vi "Get Graph Data.vi"(0 "refresh time (ms)":i32, 1 "reading.var 1::1":dbl caption="Regen pulse energy" min=-100000.0 max=100000.0, 2 "Number of hours in buffer":dbl=96.0, 3 "MeanCounts::2":dbl caption="LM_Mirrorcam MeanCounts" min=0.0 max=999999999.0, 4 "MeanCounts::3":dbl caption="LM_Focuscam MeanCounts" min=0.0 max=999999999.0, 5 "MeanCounts::4":dbl caption="TS-253a_in MeanCounts" min=0.0 max=999999999.0, 6 "Data ip":T1) -> (14 "Data op":T1, 15 "Current array size":i32)   [LabVIEW 2013]
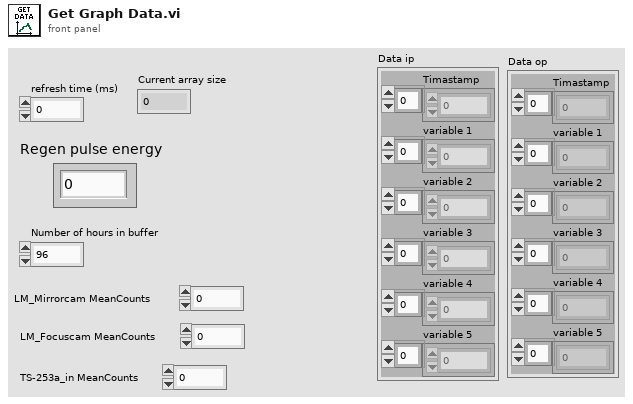
[diagram p1: front panel]
types:
  T1 = cluster{"Timastamp":dbl[], "variable 1":dbl[], "variable 2":dbl[], "variable 3":dbl[], "variable 4":dbl[], "variable 5":dbl[]}
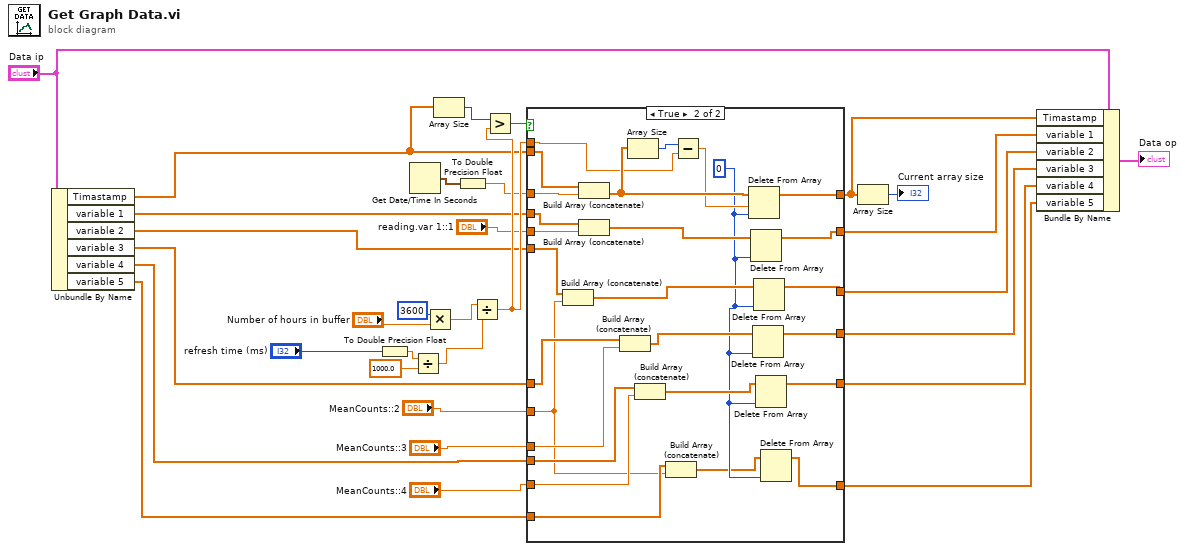
[diagram p0: block diagram]
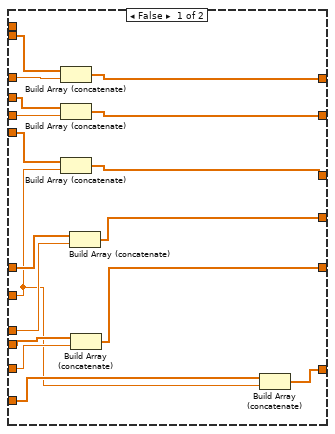
[diagram p2: hidden frame]
diagram:
  n1 = Unbundle By Name("Data ip") -> ("Timastamp"=w14:dbl[], "variable 1"=w13:dbl[], "variable 2"=w12:dbl[], "variable 3"=w11:dbl[], "variable 4"=w10:dbl[], "variable 5"=w9:dbl[])
  n2 = To Double Precision Float(number="refresh time (ms)") -> (double precision float=w22:dbl)
  n3 = Get Date/Time In Seconds() -> (seconds since 1Jan1904=w16:timestamp)
  n4 = Divide(x=w22, y=1000.0) -> (x/y=w26:dbl)
  n5 = Multiply(x=3600, y="Number of hours in buffer") -> (x*y=w25:dbl)
  n6 = Array Size(array=w14) -> (size(s)=w15:i32)
  n7 = To Double Precision Float(number=w16) -> (double precision float=w18:dbl)
  n8 = Divide(x=w25, y=w26) -> (x/y=w28:dbl)
  n9 = Greater?(x=w15, y=w28) -> (0:w17:bool)
  n10 = case shown="True" w17 {
    tunnel: w18 -> [w48 w75]
    tunnel: "reading.var 1::1" -> [w45 w74]
    tunnel: [w47 w70] -> w7
    tunnel: [w46 w69] -> w6
    tunnel: w14 -> [w44 w73]
    tunnel: w13 -> [w43 w72]
    tunnel: w28 -> [_ w66]
    tunnel: "MeanCounts::2" -> [w32 w49]
    tunnel: w12 -> [w42 w63]
    tunnel: [w41 w62] -> w5
    tunnel: "MeanCounts::3" -> [w38 w59]
    tunnel: "MeanCounts::4" -> [w34 w58]
    tunnel: [w40 w57] -> w4
    tunnel: [w39 w56] -> w3
    tunnel: w10 -> [w37 w55]
    tunnel: w11 -> [w36 w54]
    tunnel: w9 -> [w35 w50]
    tunnel: [w33 w52] -> w2
    frame False {
      n11 = Build Array (concatenate)(w44, w48) -> (w47:dbl[])
      n12 = Build Array (concatenate)(w43, w45) -> (w46:dbl[])
      n13 = Build Array (concatenate)(w42, w32) -> (w41:dbl[])
      n14 = Build Array (concatenate)(w36, w38) -> (w40:dbl[])
      n15 = Build Array (concatenate)(w37, w34) -> (w39:dbl[])
      n16 = Build Array (concatenate)(w35, w32) -> (w33:dbl[])
    }
    frame True {
      w53 = 0
      n17 = Build Array (concatenate)(w63, w49) -> (w64:dbl[])
      n18 = Build Array (concatenate)(w73, w75) -> (w68:dbl[])
      n19 = Build Array (concatenate)(w72, w74) -> (w71:dbl[])
      n20 = Build Array (concatenate)(w54, w59) -> (w60:dbl[])
      n21 = Array Size(array=w68) -> (size(s)=w67:i32)
      n22 = Build Array (concatenate)(w55, w58) -> (w61:dbl[])
      n23 = Build Array (concatenate)(w50, w49) -> (w51:dbl[])
      n24 = Subtract(x=w67, y=w66) -> (x-y=w65:dbl)
      n25 = Delete From Array(array=w68, length=w65, index=w53) -> (array with subset deleted=w70:dbl[])  [unwired: 1 out]
      n26 = Delete From Array(array=w71, index=w53) -> (array with subset deleted=w69:dbl[])  [unwired: 1 in, 1 out]
      n27 = Delete From Array(array=w60, index=w53) -> (array with subset deleted=w57:dbl[])  [unwired: 1 in, 1 out]
      n28 = Delete From Array(array=w64, index=w53) -> (array with subset deleted=w62:dbl[])  [unwired: 1 in, 1 out]
      n29 = Delete From Array(array=w61, index=w53) -> (array with subset deleted=w56:dbl[])  [unwired: 1 in, 1 out]
      n30 = Delete From Array(array=w51, index=w53) -> (array with subset deleted=w52:dbl[])  [unwired: 1 in, 1 out]
    }
  }
  n31 = Array Size(array=w7) -> (size(s)=→"Current array size":i32)
  n32 = Bundle By Name(cluster="Data ip", "Timastamp"=w7, "variable 1"=w6, "variable 2"=w5, "variable 3"=w4, "variable 4"=w3, "variable 5"=w2) -> (→"Data op":T1)
